vi "Clase4.vi"() -> ()   [LabVIEW 2011]
panel:
  out "Alarma":bool
  out "Temperatura":dbl(slide) scale=0.0..100.0
  out "Cambio":string
  out "Cuarta":bool
  out "Tercera":bool
  out "Segunda":bool
  out "Primera":bool
  out "Velocidad":i32(knob) scale=0.0..180.0
  # "Elaborar un programa donde se genere la velocidad entre 1-180, luego de acuerdo a la velocidad \nque se alcance encender en que cambio se encuentra en el string indicator el cambio.\n\n1-40 primera\n41-60 segunda\n61-80 tercera\n81-180 cuarta\n\n\nSi la temperatura es mayor a 75 y la velocidad mayor a 120 encender la alarma de\ncalentamiento."
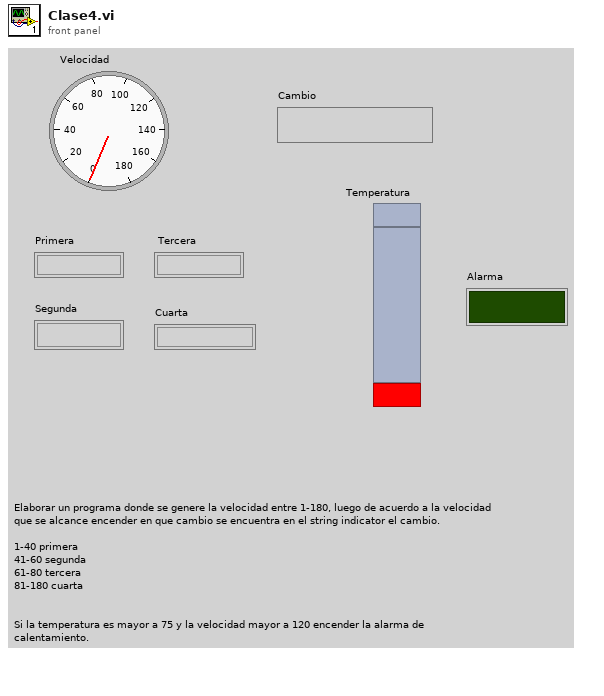
[diagram p1: front panel]
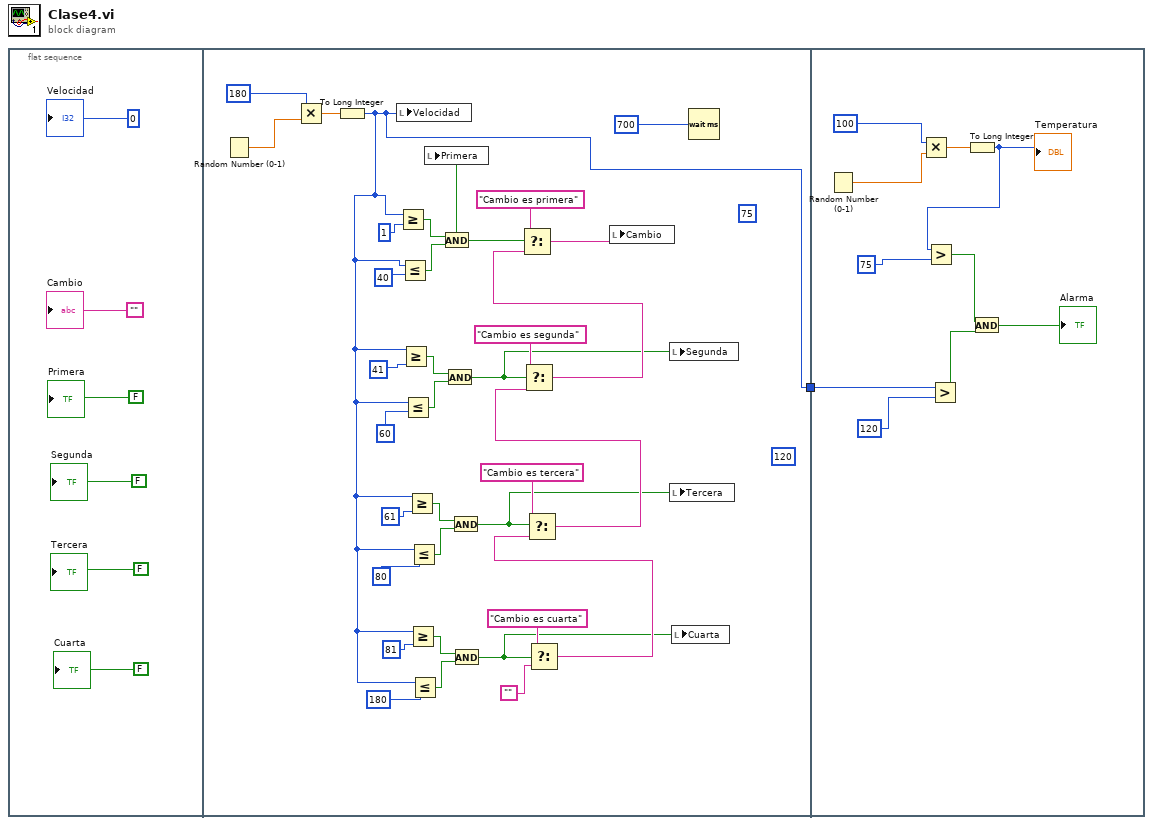
[diagram p0: block diagram]
diagram:
  n1 = flat-sequence {
    tunnel: [w8] -> w1
    tunnel: w1 -> [w45]
    frame #0 {
      "Velocidad" <- 0
      "Primera" <- FALSE
      "Segunda" <- FALSE
      "Tercera" <- FALSE
      "Cuarta" <- FALSE
      "Cambio" <- ""
    }
    frame #1 {
      (unwired) 120
      (unwired) 75
      n2 = Random Number (0-1)() -> (number: 0 to 1=w41:dbl)
      n3 = Multiply(x=180, y=w41) -> (x*y=w39:dbl)
      n4 = To Long Integer(number=w39) -> (32bit integer=w8:i32)
      n5 = local write "Velocidad"(w8) -> ()
      n6 = Greater Or Equal?(x=w8, y=1) -> (x >= y?=w36:bool)
      n7 = Less Or Equal?(x=w8, y=40 ("x")) -> (x <= y?=w35:bool)
      n8 = Greater Or Equal?(x=w8, y=41) -> (x >= y?=w30:bool)
      n9 = Less Or Equal?(x=w8, y=60 ("x")) -> (x <= y?=w31:bool)
      n10 = Greater Or Equal?(x=w8, y=61) -> (x >= y?=w23:bool)
      n11 = Greater Or Equal?(x=w8, y=81) -> (x >= y?=w18:bool)
      n12 = Less Or Equal?(x=w8, y=80 ("x")) -> (x <= y?=w22:bool)
      n13 = Less Or Equal?(x=w8, y=180 ("x")) -> (x <= y?=w19:bool)
      n14 = And(x=w36, y=w35) -> (x .and. y?=w32:bool)
      n15 = local write "Primera"(w32) -> ()
      n16 = And(x=w30, y=w31) -> (x .and. y?=w12:bool)
      n17 = And(x=w23, y=w22) -> (x .and. y?=w11:bool)
      n18 = And(x=w18, y=w19) -> (x .and. y?=w10:bool)
      n19 = Select(t="Cambio es cuarta", s=w10, f="") -> (s? t:f=w14:string)
      n20 = Select(t="Cambio es tercera", s=w11, f=w14) -> (s? t:f=w20:string)
      n21 = Select(t="Cambio es segunda", s=w12, f=w20) -> (s? t:f=w26:string)
      n22 = Select(t="Cambio es primera", s=w32, f=w26) -> (s? t:f=w33:string)
      n23 = local write "Cambio"(w33) -> ()
      n24 = local write "Segunda"(w12) -> ()
      n25 = local write "Tercera"(w11) -> ()
      n26 = local write "Cuarta"(w10) -> ()
      n27 = Wait (ms)(milliseconds to wait=700) -> ()  [unwired: 1 out]
    }
    frame #2 {
      n28 = Random Number (0-1)() -> (number: 0 to 1=w50:dbl)
      n29 = Multiply(x=100, y=w50) -> (x*y=w49:dbl)
      n30 = Greater?(x=w45, y=120) -> (0:w46:bool)
      n31 = To Long Integer(number=w49) -> (32bit integer=w42:i32)
      "Temperatura" <- w42
      n32 = Greater?(x=w42, y=75) -> (0:w47:bool)
      n33 = And(x=w47, y=w46) -> (x .and. y?=→"Alarma":bool)
    }
  }
